vi "Default Instance.vi"(10 "Instance":refnum<class>) -> (2 "Default Instance":refnum<class>)   [LabVIEW 2025, in "jettl.lvlib"]
uses:
  jettl.lvlib
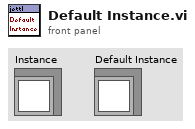
[diagram p1: front panel]
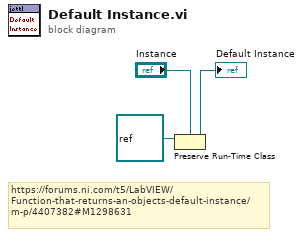
[diagram p0: block diagram]
diagram:
  # "https://forums.ni.com/t5/LabVIEW/Function-that-returns-an-objects-default-instance/m-p/4407382#M1298631"
  n1 = Preserve Run-Time Class(object in=refnum<class> refnum ("LabVIEW Object"), 2:"Instance") -> (object out=→"Default Instance":refnum<class>)  [unwired: 1 in, 1 out]
